vi "Play.vi"(8 "error in (no error)":errorcluster, 9 "fileName":string, 10 "audioType":string, 11 "MediaPlayer in":refnum<class "MediaPlayer.lvclass">) -> (0 "error out":errorcluster, 3 "MediaPlayer out":refnum<class "MediaPlayer.lvclass">)   [LabVIEW 2016, in "MediaPlayer.lvclass"]
uses:
  MediaPlayer.lvclass
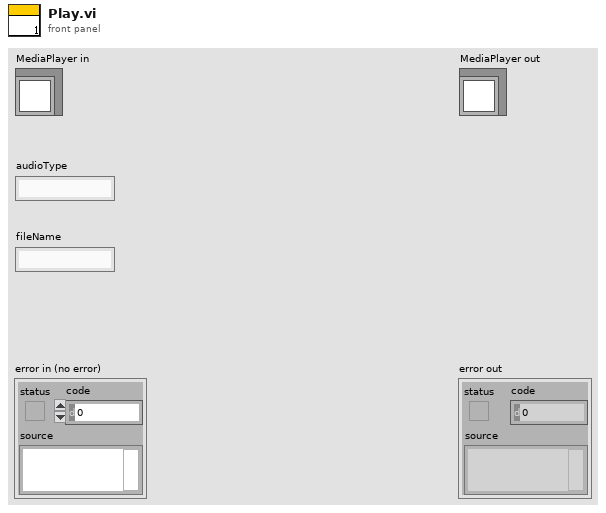
[diagram p1: front panel]
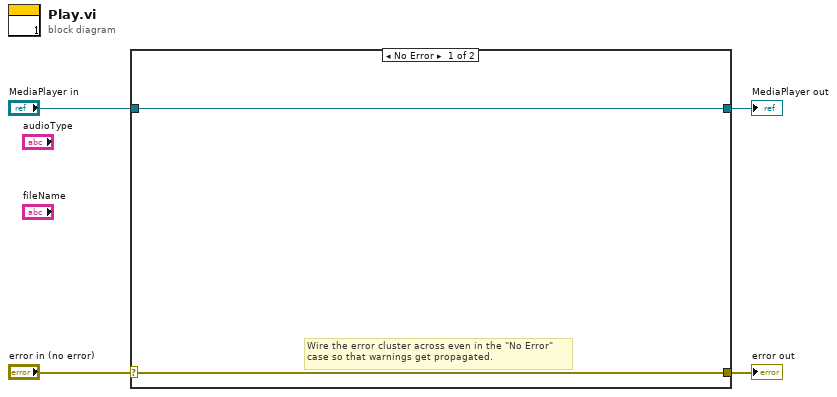
[diagram p0: block diagram]
diagram:
  n1 = case shown="No Error" "error in (no error)" {
    selector: "error in (no error)" -> [w5 w8]
    tunnel: [w5 w8] -> w3
    tunnel: [w6 w7] -> w1
    tunnel: "MediaPlayer in" -> [w6 w7]
    frame No Error {
      # "Wire the error cluster across even in the \"No Error\"\ncase so that warnings get propagated."
    }
    frame Error {
    }
  }
  "error out" <- w3
  "MediaPlayer out" <- w1
